vi "sendCMD.vi"(6 "Unit":string=" ", 8 "error in (no error)":errorcluster, 9 "Value":i32=-99999, 10 "Command":string, 11 "VISA resource name":refnum<visa-resource-name>) -> (0 "error out":errorcluster, 1 "Success?":bool=TRUE, 3 "VISA resource name out":refnum<visa-resource-name>)   [LabVIEW 2017, in "LIAinteraction.lvlib"]
uses:
  LIAinteraction.lvlib
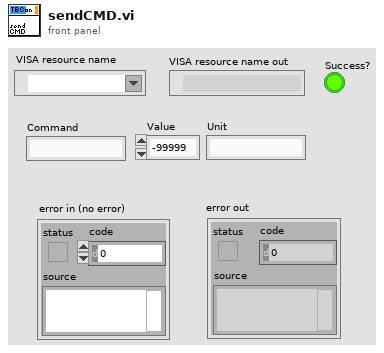
[diagram p1: front panel]
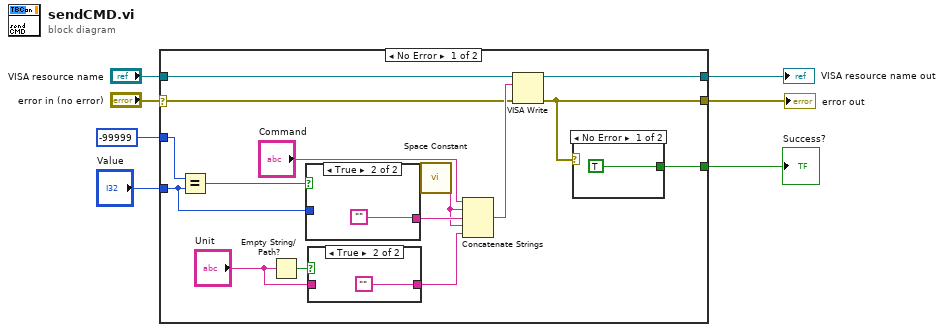
[diagram p0: block diagram]
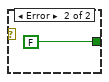
[diagram p3: hidden frame]
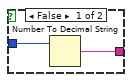
[diagram p4: hidden frame]
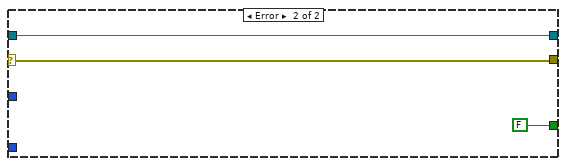
[diagram p5: hidden frame]
diagram:
  n1 = case shown="No Error" "error in (no error)" {
    selector: "error in (no error)" -> [w8 w32]
    tunnel: [w18 w31] -> w7
    tunnel: "VISA resource name" -> [w17 w31]
    tunnel: [w16 w32] -> w5
    tunnel: [w15 FALSE] -> w4
    tunnel: "Value" -> [w13 _]
    tunnel: -99999 -> [w12 _]
    frame No Error {
      n2 = Equal?(x=w12, y=w13) -> (x = y?=w14:bool)
      n3 = Empty String/Path?(string/path="Unit") -> (empty?=w11:bool)
      n4 = case shown="True" w14 {
        tunnel: w13 -> [w28 _]
        tunnel: [w27 ""] -> w22
        frame False {
          n5 = Number To Decimal String(number=w28) -> (decimal integer string=w27:string)  [unwired: 1 in]
        }
        frame True {
        }
      }
      n6 = case shown="True" w11 {
        tunnel: [w23 ""] -> w10
        tunnel: "Unit" -> [w23 _]
        frame False {
        }
        frame True {
        }
      }
      n7 = call <vilib>:"Space Constant.vi"() -> ("String"=w21:string)
      n8 = Concatenate Strings("Command", w21, w22, w21, w10) -> (w19:string)
      n9 = VISA Write(VISA resource name=w17, write buffer=w19, error in (no error)=w8) -> (VISA resource name out=w18:refnum<visa-resource-name>, error out=w16:errorcluster)  [unwired: 1 out]
      n10 = case shown="No Error" w16 {
        tunnel: [TRUE FALSE] -> w15
        frame No Error {
        }
        frame Error {
        }
      }
    }
    frame Error {
    }
  }
  "VISA resource name out" <- w7
  "error out" <- w5
  "Success?" <- w4
